vi "Pre Launch Init.vi"(11 "Supervisor in":refnum<class "Supervisor.lvclass">) -> (0 "error out":errorcluster, 3 "Supervisor out":refnum<class "Supervisor.lvclass">)   [LabVIEW 2020, in "Supervisor.lvlib" / "Supervisor.lvclass"]
doc: "<p>(<strong>Filename</strong>: <span class=\"dnl\">Actor Framework.lvlib:Actor.lvclass:Pre Launch Init.vi</span>)</p>\n<p>Defines behavior that occurs after the <a href=\"nihelplauncher://docs/csh?context=lvcore_lvcomm_af_launch_nested_actor\">Launch Nested Actor</a> method is invoked but before the actor's Actor Core method begins running.</p>\n<p>By default, this method does nothing. A descendant class may override it to define behavior.</p>"
uses:
  Supervisor.lvclass
  Supervisor.lvclass/Supervisor.ctl
  <vilib>/ActorFramework/Actor/Actor.lvclass
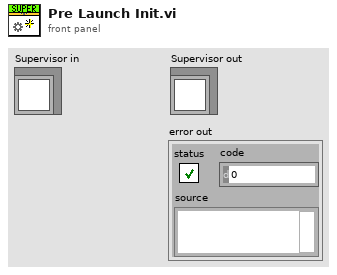
[diagram p1: front panel]
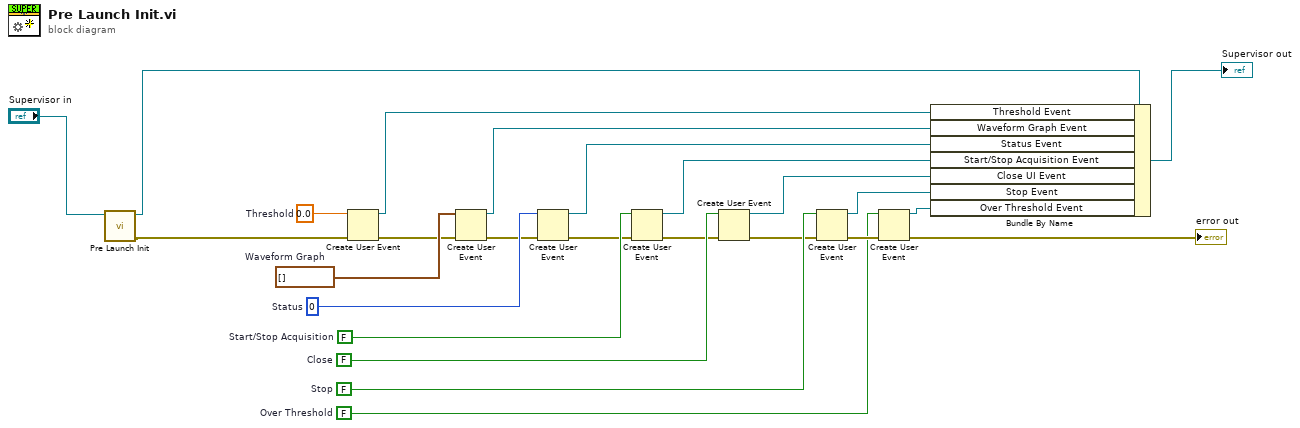
[diagram p0: block diagram]
diagram:
  w3 = FALSE  # Over Threshold
  w7 = FALSE  # Stop
  w10 = FALSE  # Close
  w13 = FALSE  # Start/Stop Acquisition
  w17 = 0.0  # Threshold
  w21 = waveform(dbl)[] []  # Waveform Graph
  w22 = u8 0  # Status
  n1 = call-parent "Pre Launch Init.vi"("Actor in"="Supervisor in") -> ("error out"=w20:errorcluster, "Actor out"=w24:refnum<class "Supervisor.lvclass">)  [unwired: 9 in]
  n2 = Create User Event(user event datatype=w17, error in=w20) -> (user event=w16:refnum<user-event>, error out=w14:errorcluster)
  n3 = Create User Event(user event datatype=w21, error in=w14) -> (user event=w19:refnum<user-event>, error out=w15:errorcluster)
  n4 = Create User Event(user event datatype=w22, error in=w15) -> (user event=w18:refnum<user-event>, error out=w12:errorcluster)
  n5 = Create User Event(user event datatype=w13, error in=w12) -> (user event=w11:refnum<user-event>, error out=w9:errorcluster)
  n6 = Create User Event(user event datatype=w10, error in=w9) -> (user event=w8:refnum<user-event>, error out=w6:errorcluster)
  n7 = Create User Event(user event datatype=w7, error in=w6) -> (user event=w5:refnum<user-event>, error out=w4:errorcluster)
  n8 = Create User Event(user event datatype=w3, error in=w4) -> (user event=w2:refnum<user-event>, error out=→"error out":errorcluster)
  n9 = Bundle By Name(cluster=w24, "Threshold Event"=w16, "Waveform Graph Event"=w19, "Status Event"=w18, "Start/Stop Acquisition Event"=w11, "Close UI Event"=w8, "Stop Event"=w5, "Over Threshold Event"=w2) -> (→"Supervisor out":refnum<class "Supervisor.lvclass">)
